vi "Increment.vi"(8 "error in (no error)":errorcluster, 11 "Standard in":refnum<class "Standard.lvclass">) -> (0 "error out":errorcluster, 3 "Standard out":refnum<class "Standard.lvclass">)   [LabVIEW 2020, in "Standard.lvclass"]
uses:
  Standard.lvclass
  Counter/Counter.lvclass
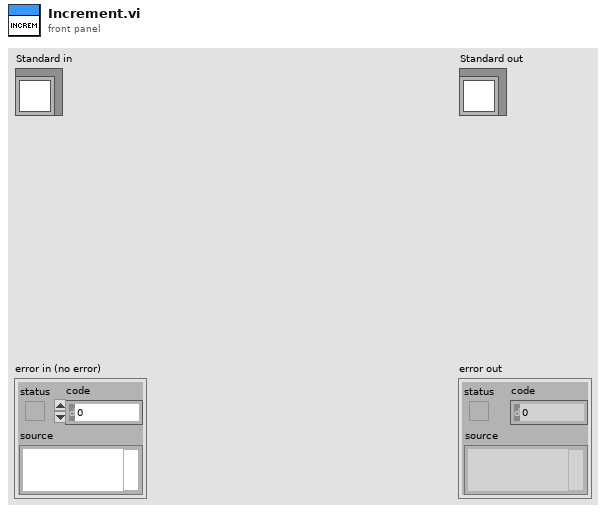
[diagram p1: front panel]
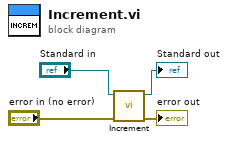
[diagram p0: block diagram]
diagram:
  n1 = call-parent "Increment.vi"("error in (no error)"="error in (no error)", "Counter in"="Standard in") -> ("error out"=→"error out":errorcluster, "Counter out"=→"Standard out":refnum<class "Standard.lvclass">)  [unwired: 8 in]
